vi "PythontoArray.vi"(8 "error in (no error)":errorcluster, 10 "command line":string="python SkysparkBuild3.py", 11 "working directory":path=path "") -> (0 "error out":errorcluster, 2 "standard output":string, 3 "Output Array":string[][](array[string]))   [LabVIEW 2020]
uses:
  859b58b0-79df-43f2-a2e9-99a1650faf3a.vi
panel:
  out "Table Control":string[][](table)
  in  "format string":string
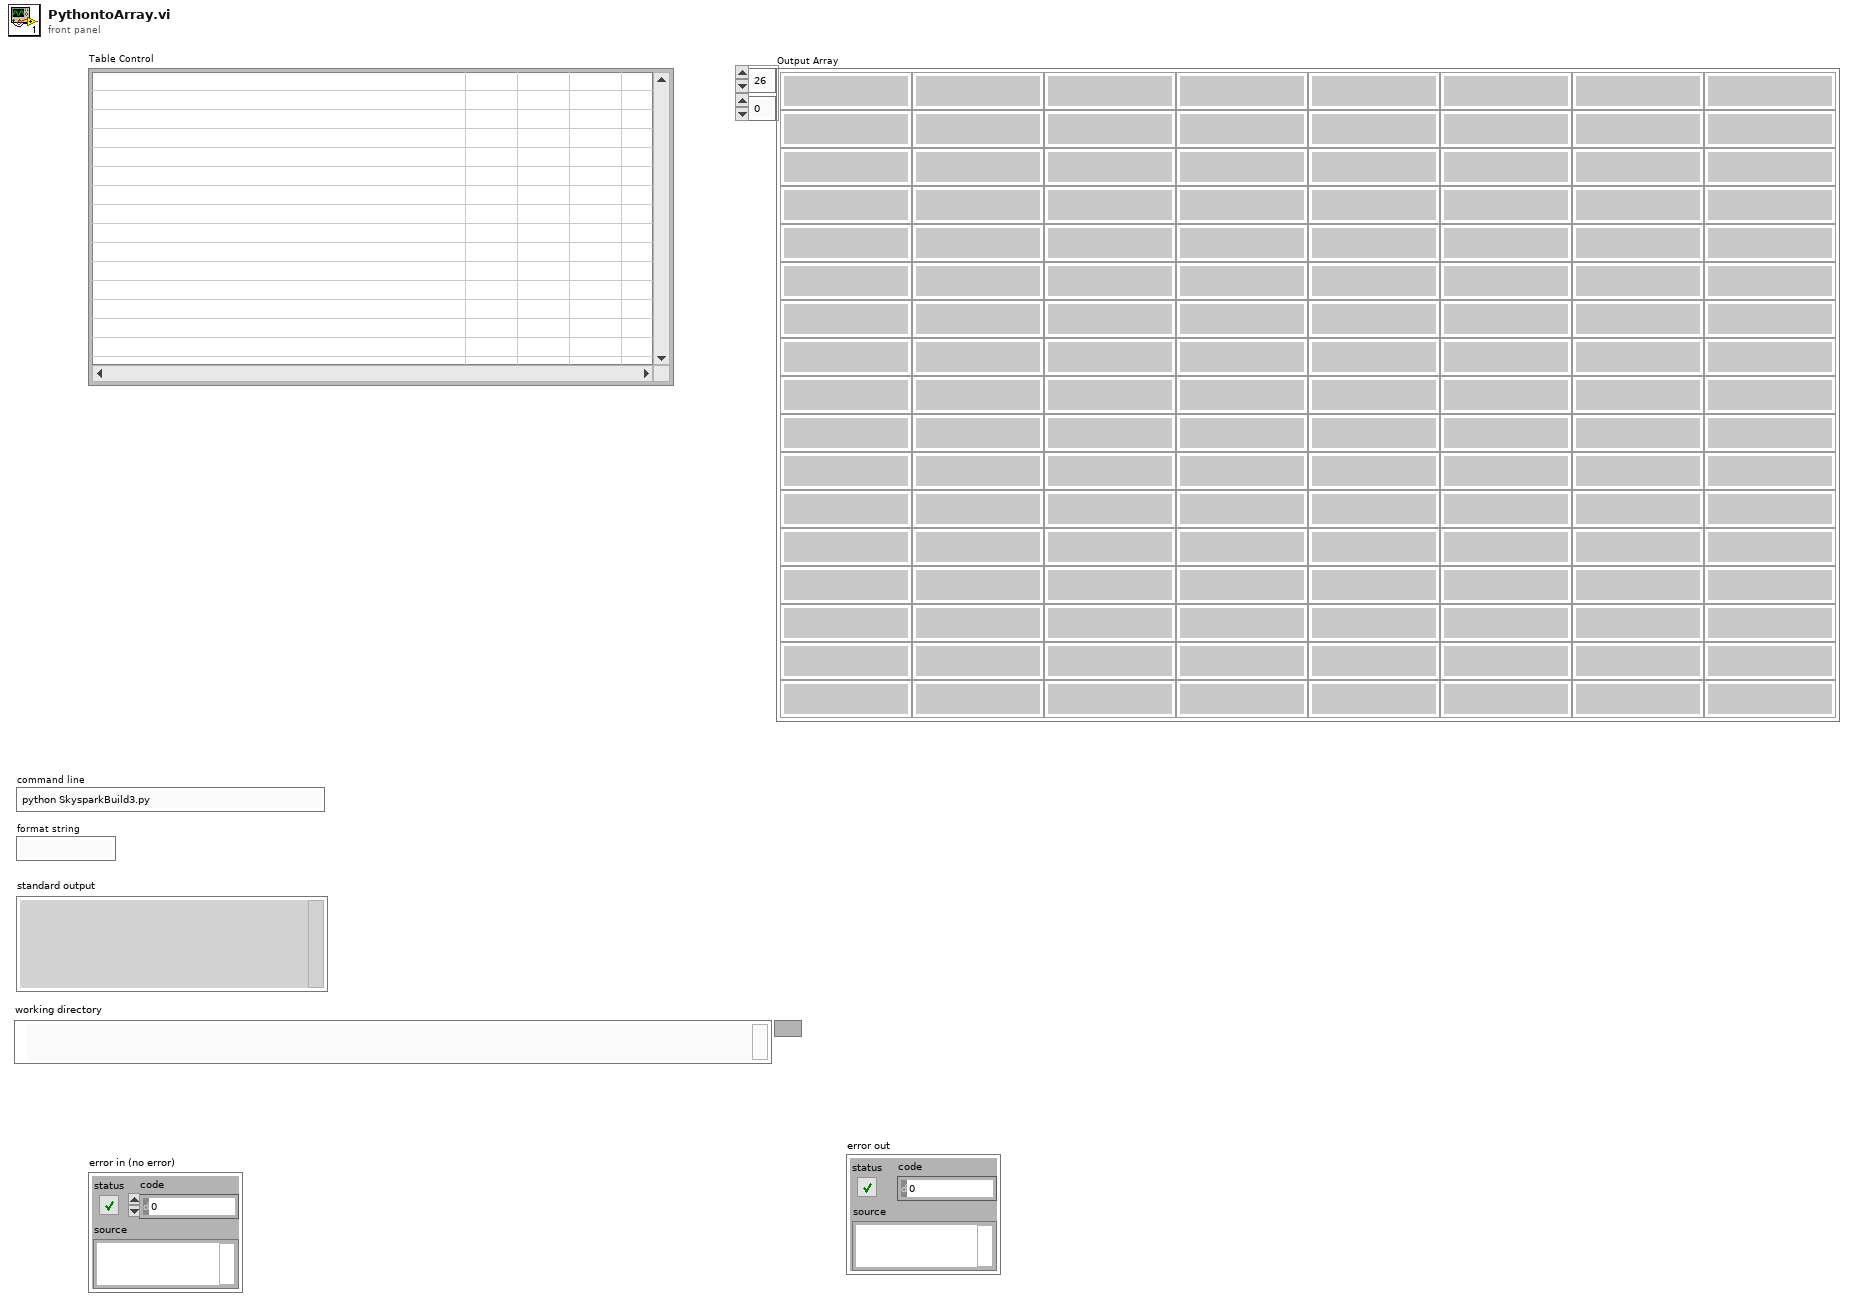
[diagram p1: front panel]
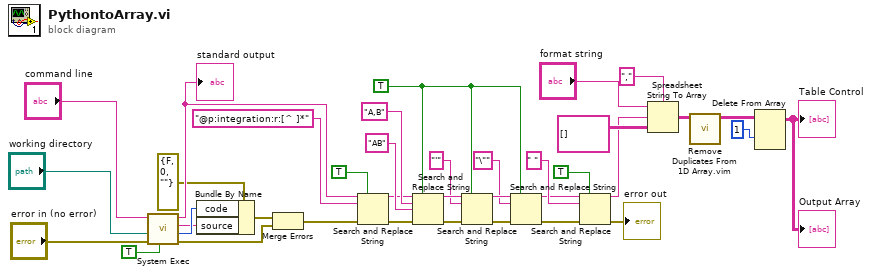
[diagram p0: block diagram]
diagram:
  w19 = TRUE ("replace all? (F)")
  n1 = call "System Exec.vi"("run minimized? (F)"=TRUE, "error in (no error)"="error in (no error)", "working directory"="working directory", "command line"="command line") -> ("error out"=w6:errorcluster, "return code"=w3:i32, "standard error"=w1:string, "standard output"=w23:string)  [unwired: 4 in]
  "standard output" <- w23
  n2 = Bundle By Name(cluster=errorcluster {"status"=FALSE, "code"=0, "source"=""} ("error in"), "code"=w3, "source"=w1) -> (w2:errorcluster)
  n3 = Merge Errors(w2, w6) -> (w5:errorcluster)
  n4 = Search and Replace String(replace all?=TRUE ("replace all? (F)"), input string=w23, search string="@p:integration:r:[^ ]*", error in=w5) -> (result string=w24:string, error out=w15:errorcluster)  [unwired: 4 in, 2 out]
  n5 = Search and Replace String(replace all?=w19, input string=w24, search string="A,B" ("substring (\"\")"), replace string="AB" ("replace string (\"\")"), error in=w15) -> (result string=w22:string, error out=w14:errorcluster)  [unwired: 3 in, 2 out]
  n6 = Search and Replace String(replace all?=w19, input string=w22, search string="'", error in=w14) -> (result string=w21:string, error out=w20:errorcluster)  [unwired: 4 in, 2 out]
  n7 = Search and Replace String(replace all?=w19, input string=w21, search string="\"", error in=w20) -> (result string=w9:string, error out=w12:errorcluster)  [unwired: 4 in, 2 out]
  n8 = Search and Replace String(replace all?=TRUE ("replace all? (F)"), input string=w9, search string=" ", error in=w12) -> (result string=w8:string, error out=→"error out":errorcluster)  [unwired: 4 in, 2 out]
  n9 = Spreadsheet String To Array(delimiter (Tab)=",", format string="format string", spreadsheet string=w8, array type (2D Dbl)=string[][] []) -> (array=w31:string[][])
  n10 = call "Remove Duplicates From 1D Array.vim"("array"=w31) -> ("array with duplicates removed"=w30:string[][])  [unwired: 10 in]
  n11 = Delete From Array(array=w30, index (row)=1) -> (array with subset deleted=→"Output Array" →"Table Control":string[][])  [unwired: 2 in, 1 out]
